vi "Main.vi"() -> ()   [LabVIEW 2015]
uses:
  <vilib>/ActorFramework/Actor/Actor.lvclass
  Example Source/Example Source/Example Source.lvclass
  Example Sink/Example Sink/Example Sink.lvclass
  Event Source/Event Source Messages/Register Msg/Register Msg.lvclass
  Example Source/Example Events/Double Array Event.lvclass
  Example Source/Example Events/Timestamp Event.lvclass
  Example Sink/Example Sink Messages/Update Time Msg/Update Time Msg.lvclass
  Example Sink/Example Sink Messages/Update Array Msg/Update Array Msg.lvclass
  Timed Loop Controller/Timed Loop Controller/Timed Loop Controller.lvclass
  <vilib>/ActorFramework/Stop Msg/Stop Msg.lvclass
  Event Source/Event Source Messages/Unregister Msg/Unregister Msg.lvclass
  Event Source/Event Source Messages/Unregister Event Msg/Unregister Event Msg.lvclass
  Event Source/Event/Event.lvclass
panel:
  in  "Registered for Data":bool
  in  "Registered for Time":bool
  in  "Stop Button":bool
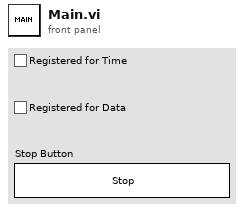
[diagram p1: front panel]
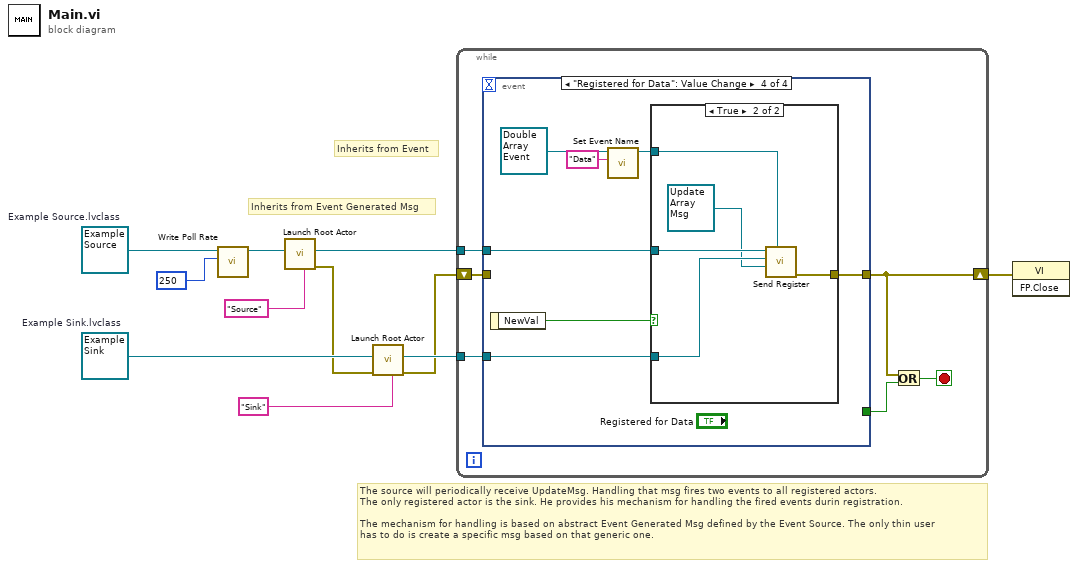
[diagram p0: block diagram]
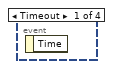
[diagram p2: hidden frame]
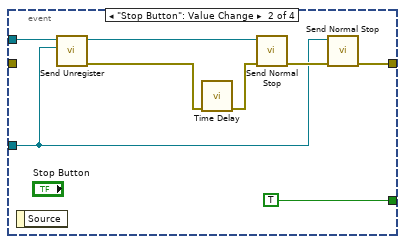
[diagram p3: hidden frame]
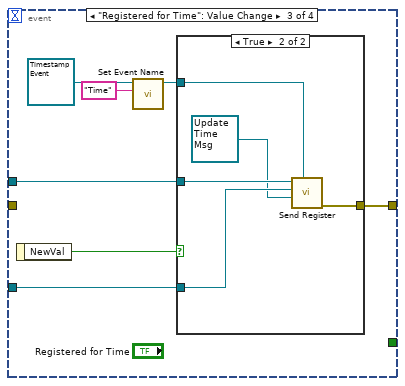
[diagram p4: hidden frame]
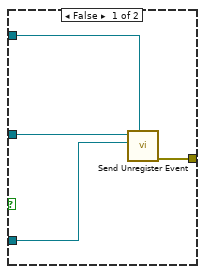
[diagram p5: hidden frame]
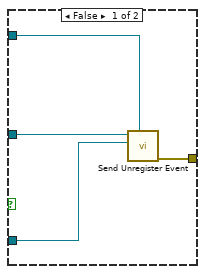
[diagram p6: hidden frame]
diagram:
  w11 = refnum<class "Example Sink.lvclass"> refnum  # Example Sink.lvclass
  w10 = refnum<class "Example Source.lvclass"> refnum  # Example Source.lvclass
  # "The source will periodically receive UpdateMsg. Handling that msg fires two events to all registered actors.\nThe only registered actor is the sink. He provides his mechanism for handling the fired events durin registration.\n\nThe mechanism for handling is based on abstract Event Generated Msg defined by the Event Source. The only thin user\nhas to do is create a specific msg based on that generic one."
  # "Inherits from Event"
  # "Inherits from Event Generated Msg"
  n1 = call "Write Poll Rate.vi"("Poll Rate"=u32 250, "Timed Loop Controller in"=w10) -> ("Timed Loop Controller out"=w9:refnum<class "Example Source.lvclass">)  [unwired: 8 in, 1 out]
  n2 = call <vilib>:"Launch Root Actor.vi"("Debug Alias"="Source", "Actor"=w9) -> ("error out"=w4:errorcluster, "Actor's Enqueuer"=w5:refnum<class "Message Enqueuer.lvclass">)  [unwired: 8 in]
  n3 = call <vilib>:"Launch Root Actor.vi"("Debug Alias"="Sink", "error in (no error)"=w4, "Actor"=w11) -> ("error out"=w3:errorcluster, "Actor's Enqueuer"=w6:refnum<class "Message Enqueuer.lvclass">)  [unwired: 7 in]
  n4 = while {
    tunnel: w5 -> [w16]
    tunnel: w6 -> [w15]
    shift-right: [w13] -> w7
    shift-left: w3 -> [w17]
    stop <- w12 stop-if-true
    n5 = event shown="[3] \"Registered for Data\": Value Change" {
      selector: _ -> [_ _ _ _]
      dyn-events: _ -> [_ _ _ _]
      timeout: _ -> [_ _ _ _]
      tunnel: w17 -> [_ _ _ _]
      tunnel: w16 -> [_ w24 w31 w47]
      tunnel: w15 -> [_ w20 w30 w46]
      tunnel: [_ w19 w29 w45] -> w13
      tunnel: [_ TRUE _ _] -> w14
      event Timeout {
        n6 = event-data() -> ()  [unwired: 1 in, 1 out]
      }
      event "Stop Button": Value Change {
        n7 = event-data() -> ()  [unwired: 1 in, 1 out]
        n8 = call "Send Unregister.vi"("Registrant Address"=w20, "Event Source Address"=w24) -> ("Error Out"=w22:errorcluster, "Event Source Address Out"=w23:refnum<class "Message Enqueuer.lvclass">)  [unwired: 8 in]
        n9 = call "Time Delay"("error in (no error)"=w22) -> ("error out"=w21:errorcluster)  [unwired: 10 in]
        n10 = call <vilib>:"Send Normal Stop.vi"("error in (no error)"=w21, "Message Enqueuer"=w23) -> ("error out"=w25:errorcluster)  [unwired: 9 in]
        n11 = call <vilib>:"Send Normal Stop.vi"("error in (no error)"=w25, "Message Enqueuer"=w20) -> ("error out"=w19:errorcluster)  [unwired: 9 in]
      }
      event "Registered for Time": Value Change {
        n12 = event-data() -> ("NewVal"=w32:bool)  [unwired: 1 in]
        n13 = call "Set Event Name.vi"("Name (Generic)"="Time", "Event In"=refnum<class "Timestamp Event.lvclass"> refnum ("Timestamp Event.lvclass")) -> ("Event Out"=w26:refnum<class "Timestamp Event.lvclass">)  [unwired: 9 in]
        n14 = case shown="True" w32 {
          tunnel: w31 -> [w36 w41]
          tunnel: w30 -> [w34 w40]
          tunnel: w26 -> [w35 w38]
          tunnel: [w33 w37] -> w29
          frame False {
            n15 = call "Send Unregister Event.vi"("Event"=w35, "Registrant Address"=w34, "Event Source Address"=w36) -> ("Error Out"=w33:errorcluster)  [unwired: 7 in, 1 out]
          }
          frame True {
            n16 = call "Send Register.vi"("Event"=w38, "Event Handler"=refnum<class "Update Time Msg.lvclass"> refnum ("Update Time Msg.lvclass"), "Registrant Address"=w40, "Event Source Address"=w41) -> ("Error Out"=w37:errorcluster)  [unwired: 6 in, 1 out]
          }
        }
      }
      event "Registered for Data": Value Change {
        n17 = event-data() -> ("NewVal"=w48:bool)  [unwired: 1 in]
        n18 = call "Set Event Name.vi"("Name (Generic)"="Data", "Event In"=refnum<class "Double Array Event.lvclass"> refnum ("Double Array Event.lvclass")) -> ("Event Out"=w43:refnum<class "Double Array Event.lvclass">)  [unwired: 9 in]
        n19 = case shown="True" w48 {
          tunnel: w47 -> [w52 w57]
          tunnel: w46 -> [w50 w56]
          tunnel: w43 -> [w51 w55]
          tunnel: [w49 w54] -> w45
          frame False {
            n20 = call "Send Unregister Event.vi"("Event"=w51, "Registrant Address"=w50, "Event Source Address"=w52) -> ("Error Out"=w49:errorcluster)  [unwired: 7 in, 1 out]
          }
          frame True {
            n21 = call "Send Register.vi"("Event"=w55, "Event Handler"=refnum<class "Update Array Msg.lvclass"> refnum ("Update Array Msg.lvclass"), "Registrant Address"=w56, "Event Source Address"=w57) -> ("Error Out"=w54:errorcluster)  [unwired: 6 in, 1 out]
          }
        }
      }
    }
    n22 = Or(x=w13, y=w14) -> (x .or. y?=w12:bool)
  }
  n23 = invoke class="VI" method="FP.Close"(error in=w7) -> ()  [unwired: 2 in, 3 out]
